vi "output_current_to_flow.vi"(1 "Output Current":dbl[](array[numeric])) -> (0 "Flow rate":dbl)   [LabVIEW 2015]
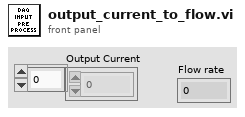
[diagram p1: front panel]
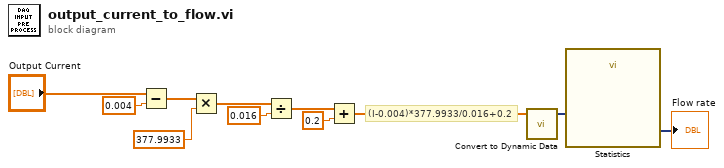
[diagram p0: block diagram]
diagram:
  # "(I-0.004)*377.9933/0.016+0.2"
  n1 = Subtract(x="Output Current", y=0.004) -> (x-y=w9:dbl[])
  n2 = Multiply(x=w9, y=377.9933) -> (x*y=w7:dbl[])
  n3 = Divide(x=w7, y=0.016) -> (x/y=w5:dbl[])
  n4 = Add(x=w5, y=0.2) -> (x+y=w3:dbl[])
  n5 = call "Convert to Dynamic Data"("Array"=w3) -> ("Dynamic Data Type"=w2:dynamicdata)  [unwired: 3 in]
  n6 = call "Statistics"("Signals"=w2) -> ("Arithmetic Mean"=→"Flow rate":dynamicdata)  [unwired: 25 in, 1 out]
